vi "CmdControlP.vi"(3 "Type 10_F":bool) -> (1 "Dataout":u8[](array[numeric]))   [LabVIEW 2017]
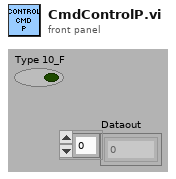
[diagram p1: front panel]
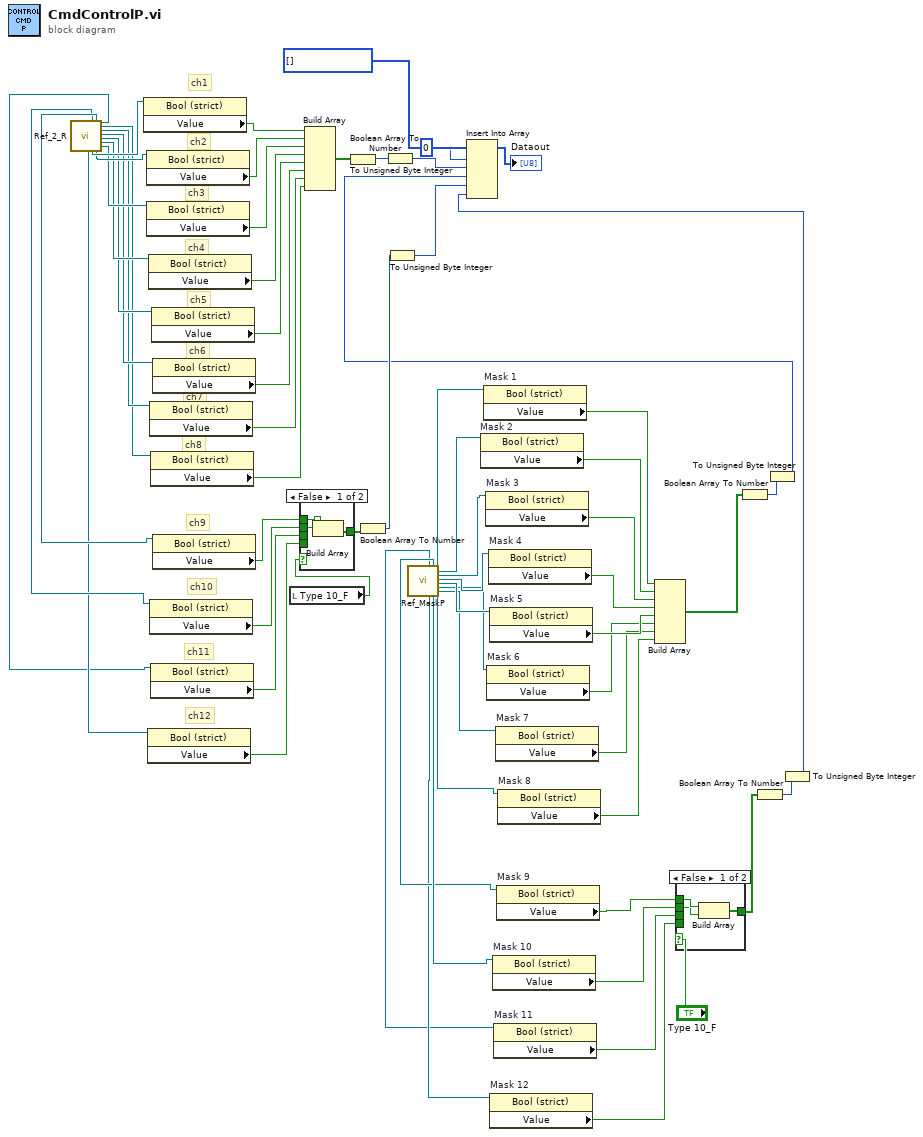
[diagram p0: block diagram]
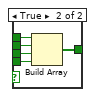
[diagram p2: hidden frame]
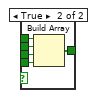
[diagram p3: hidden frame]
diagram:
  # "ch12"
  # "ch11"
  # "ch10"
  # "ch9"
  # "ch8"
  # "ch7"
  # "ch6"
  # "ch5"
  # "ch4"
  # "ch3"
  # "ch2"
  # "ch1"
  n1 = call "Ref_2_R.vi"() -> ("Control  Ch 12 out"=w8:refnum<vi>, "Control  Ch 10 out"=w42:refnum<vi>, "Control  Ch 1 out"=w63:refnum<vi>, "Control  Ch 9 out"=w43:refnum<vi>, "Control  Ch 2 out"=w62:refnum<vi>, "Control  Ch 11 out"=w7:refnum<vi>, "Control  Ch 8 out"=w56:refnum<vi>, "Control  Ch 7 out"=w57:refnum<vi>, "Control  Ch 6 out"=w58:refnum<vi>, "Control  Ch 5 out"=w59:refnum<vi>, "Control  Ch 4 out"=w60:refnum<vi>, "Control  Ch 3 out"=w61:refnum<vi>)  [unwired: 15 in, 1 out]
  n2 = property class="Bool (strict)"(reference=w63) -> ("Value"=w55:bool)  [unwired: 1 in, 2 out]
  n3 = property class="Bool (strict)"(reference=w62) -> ("Value"=w54:bool)  [unwired: 1 in, 2 out]
  n4 = property class="Bool (strict)"(reference=w61) -> ("Value"=w53:bool)  [unwired: 1 in, 2 out]
  n5 = property class="Bool (strict)"(reference=w8) -> ("Value"=w9:bool)  [unwired: 1 in, 2 out]
  n6 = property class="Bool (strict)"(reference=w60) -> ("Value"=w52:bool)  [unwired: 1 in, 2 out]
  n7 = property class="Bool (strict)"(reference=w57) -> ("Value"=w49:bool)  [unwired: 1 in, 2 out]
  n8 = property class="Bool (strict)"(reference=w42) -> ("Value"=w40:bool)  [unwired: 1 in, 2 out]
  n9 = property class="Bool (strict)"(reference=w56) -> ("Value"=w48:bool)  [unwired: 1 in, 2 out]
  n10 = property class="Bool (strict)"(reference=w7) -> ("Value"=w10:bool)  [unwired: 1 in, 2 out]
  n11 = property class="Bool (strict)"(reference=w59) -> ("Value"=w51:bool)  [unwired: 1 in, 2 out]
  n12 = property class="Bool (strict)"(reference=w58) -> ("Value"=w50:bool)  [unwired: 1 in, 2 out]
  n13 = property class="Bool (strict)"(reference=w43) -> ("Value"=w41:bool)  [unwired: 1 in, 2 out]
  n14 = local read "Type 10_F"() -> (w1:bool)
  n15 = case shown="False" w1 {
    tunnel: w41 -> [w68 w73]
    tunnel: w40 -> [w67 w72]
    tunnel: [w66 w71] -> w39
    tunnel: w10 -> [_ w70]
    tunnel: w9 -> [_ w69]
    frame False {
      n16 = Build Array(w68, w67) -> (w66:bool[])
    }
    frame True {
      n17 = Build Array(w73, w72, w70, w69) -> (w71:bool[])
    }
  }
  n18 = Build Array(w55, w54, w53, w52, w51, w50, w49, w48) -> (w47:bool[])
  n19 = Boolean Array To Number(Boolean array=w47) -> (number=w46:u32)
  n20 = Boolean Array To Number(Boolean array=w39) -> (number=w38:u32)
  n21 = To Unsigned Byte Integer(number=w46) -> (unsigned 8bit integer=w45:u8)
  n22 = To Unsigned Byte Integer(number=w38) -> (unsigned 8bit integer=w37:u8)
  n23 = call "Ref_MaskP.vi"() -> ("Mask Ch 11 out"=w3:refnum<vi>, "Mask Ch 12 out"=w4:refnum<vi>, "Mask Ch 9 out"=w17:refnum<vi>, "Mask Ch 10 out"=w18:refnum<vi>, "Mask Ch 1 out"=w26:refnum<vi>, "Mask Ch 2 out"=w25:refnum<vi>, "Mask Ch 3 out"=w24:refnum<vi>, "Mask Ch 4 out"=w23:refnum<vi>, "Mask Ch 5 out"=w22:refnum<vi>, "Mask Ch 6 out"=w21:refnum<vi>, "Mask Ch 7 out"=w20:refnum<vi>, "Mask Ch 8 out"=w19:refnum<vi>)  [unwired: 16 in]
  n24 = property on="Mask 2" class="Bool (strict)"(reference=w25) -> ("Value"=w33:bool)  [unwired: 1 in, 2 out]
  n25 = property on="Mask 1" class="Bool (strict)"(reference=w26) -> ("Value"=w34:bool)  [unwired: 1 in, 2 out]
  n26 = property on="Mask 3" class="Bool (strict)"(reference=w24) -> ("Value"=w32:bool)  [unwired: 1 in, 2 out]
  n27 = property on="Mask 6" class="Bool (strict)"(reference=w21) -> ("Value"=w29:bool)  [unwired: 1 in, 2 out]
  n28 = property on="Mask 4" class="Bool (strict)"(reference=w23) -> ("Value"=w31:bool)  [unwired: 1 in, 2 out]
  n29 = property on="Mask 5" class="Bool (strict)"(reference=w22) -> ("Value"=w30:bool)  [unwired: 1 in, 2 out]
  n30 = property on="Mask 12" class="Bool (strict)"(reference=w4) -> ("Value"=w5:bool)  [unwired: 1 in, 2 out]
  n31 = property on="Mask 10" class="Bool (strict)"(reference=w18) -> ("Value"=w13:bool)  [unwired: 1 in, 2 out]
  n32 = property on="Mask 11" class="Bool (strict)"(reference=w3) -> ("Value"=w6:bool)  [unwired: 1 in, 2 out]
  n33 = property on="Mask 7" class="Bool (strict)"(reference=w20) -> ("Value"=w28:bool)  [unwired: 1 in, 2 out]
  n34 = property on="Mask 9" class="Bool (strict)"(reference=w17) -> ("Value"=w14:bool)  [unwired: 1 in, 2 out]
  n35 = property on="Mask 8" class="Bool (strict)"(reference=w19) -> ("Value"=w27:bool)  [unwired: 1 in, 2 out]
  n36 = Build Array(w34, w33, w32, w31, w30, w29, w28, w27) -> (w35:bool[])
  n37 = case shown="False" "Type 10_F" {
    tunnel: [w74 w81] -> w15
    tunnel: w14 -> [w76 w80]
    tunnel: w13 -> [w75 w79]
    tunnel: w6 -> [_ w78]
    tunnel: w5 -> [_ w77]
    frame False {
      n38 = Build Array(w76, w75) -> (w74:bool[])
    }
    frame True {
      n39 = Build Array(w80, w79, w78, w77) -> (w81:bool[])
    }
  }
  n40 = Boolean Array To Number(Boolean array=w35) -> (number=w36:u32)
  n41 = Boolean Array To Number(Boolean array=w15) -> (number=w16:u32)
  n42 = To Unsigned Byte Integer(number=w36) -> (unsigned 8bit integer=w12:u8)
  n43 = To Unsigned Byte Integer(number=w16) -> (unsigned 8bit integer=w11:u8)
  n44 = Insert Into Array(array=u8[] [] ("Data 2"), index=0, new element #1=w45, new element #2=w12, new element #3=w37, new element #4=w11) -> (→"Dataout":u8[])
